vi "Plucker_Force_CoordTransform.vi"(9 "R_{1}_{2}":dbl[][](array[numeric]), 10 "d_{1}_{2} (mm)":dbl[](array[numeric]), 11 "F_{1}":dbl[](array[numeric])) -> (3 "F_{2}":dbl[](array[numeric]))   [LabVIEW 2019]
uses:
  <vilib>/imath/engines/lvmath2/RunTimeEngine/Managers/WorkSpace/UID Generator.vi
  <vilib>/imath/engines/lvmath2/RunTimeEngine/BuiltInFunctions/size/NIMS_[I32,I32]=size(GRow).vi
  <instcachedir>/0/NIMS_[I32,I32]=size(GRow)_CFE2C4BDC5BC45CD88F2F6A295A2273D.lvgen/NIMS_[I32,I32]=size(GRow)_CFE2C4BDC5BC45CD88F2F6A295A2273D_001.vi
  <vilib>/imath/engines/lvmath2/RunTimeEngine/RunTimeType/NIMS_RunTimeType_From StrictType (excl LVString).vi
  <instcachedir>/0/NIMS_RunTimeType_From StrictType (excl LVString)_D8AFBA86A94845AAA577C895450664BD.lvgen/NIMS_RunTimeType_From StrictType (excl LVString)_D8AFBA86A94845AAA577C895450664BD_000.vi
  <vilib>/imath/engines/lvmath2/RunTimeEngine/LocalVariableDefStatement/MC_LocalVariableDefStatement_Display.vi
  <vilib>/imath/engines/lvmath2/RunTimeEngine/IndexRead/NIMS V(S).vi
  <instcachedir>/0/NIMS V(S)_0488751826AF41519A22953C041130DC.lvgen/NIMS V(S)_0488751826AF41519A22953C041130DC_000.vi
  <vilib>/imath/engines/lvmath2/RunTimeEngine/ErrorHandling/NIMS_Create Error From Enums.vi
  <vilib>/imath/engines/lvmath2/RunTimeEngine/RowToken/NIMS_RowToken_M_M.vi
  <instcachedir>/0/NIMS_RowToken_M_M_21FE36D058524603B8B587AC30FD72C2.lvgen/NIMS_RowToken_M_M_21FE36D058524603B8B587AC30FD72C2_004.vi
  <vilib>/imath/engines/lvmath2/RunTimeEngine/ArithmeticOperatorToken/NIMS_ArithmeticOperator_multmx.vi
  <instcachedir>/0/NIMS_ArithmeticOperator_multmx_77F1D2D6F4D94BA7A97C4E7185C02392.lvgen/NIMS_ArithmeticOperator_multmx_77F1D2D6F4D94BA7A97C4E7185C02392_004.vi
  <vilib>/imath/engines/lvmath2/RunTimeEngine/MatrixToken/NIMS_MatrixToken_M_M.vi
  <instcachedir>/0/NIMS_MatrixToken_M_M_5CE23C568F32465C96BE328F7823DCA0.lvgen/NIMS_MatrixToken_M_M_5CE23C568F32465C96BE328F7823DCA0_004.vi
  <vilib>/imath/engines/lvmath2/RunTimeEngine/BuiltInFunctions/inv/NIMS_inv(GM).vi
  <instcachedir>/0/NIMS_inv(GM)_A6DF8FE880224208AACFE4CF9F659502.lvgen/NIMS_inv(GM)_A6DF8FE880224208AACFE4CF9F659502_000.vi
  <vilib>/imath/engines/lvmath2/RunTimeEngine/ErrorHandling/NIMS_Error From Error Code.vi
  <vilib>/imathl/engines/lvmath/Functions/Error Handling/Create Error.vi
  <vilib>/imath/engines/lvmath2/RunTimeEngine/Managers/SymbolTable/Clear UID.vi
  <vilib>/imath/engines/lvmath2/RunTimeEngine/NodeEndStatement/NIMS_NodeEndStatement_Output.vi
  <instcachedir>/0/NIMS_NodeEndStatement_Output_53EC0D466D134D7ABD903AC30B43404B.lvgen/NIMS_NodeEndStatement_Output_53EC0D466D134D7ABD903AC30B43404B_002.vi
  <vilib>/imath/engines/lvmath2/RunTimeEngine/ErrorHandling/NIMS_Finalize Error.vi
  <vilib>/imath/engines/lvmath2/RunTimeEngine/Managers/SymbolTable/NIMS_WorkSpace.lvlib
panel:
  out "X":dbl[][](array[numeric])
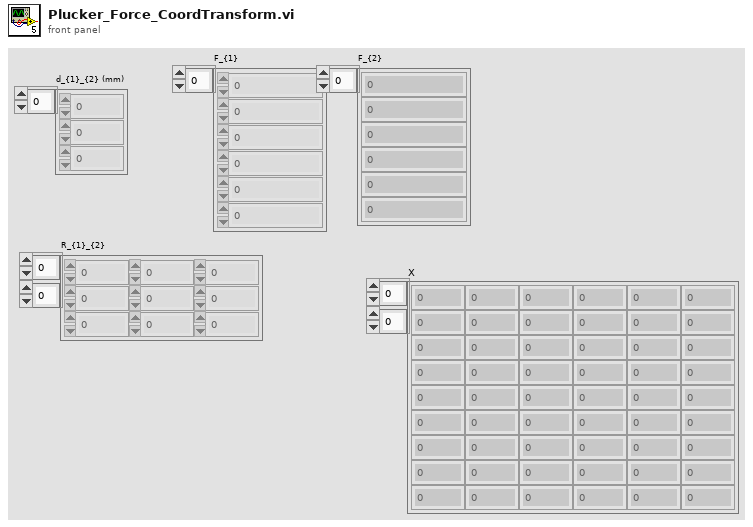
[diagram p1: front panel]
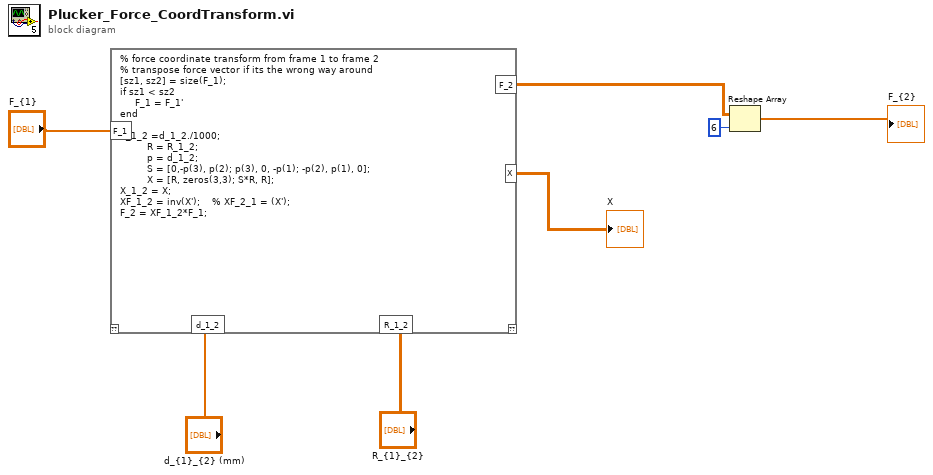
[diagram p0: block diagram]
diagram:
  n1 = mathscript code="% force coordinate transform from frame 1 to frame 2 \n% transpose force vector if its the wrong way around\n[sz1, sz2] = size(F_1);\nif sz1 < sz2\n     F_1 = F_1'\nend\n\nd_1_2 =d_1_2./1000;\n         R = R_1_2;\n         p = d_1_2;\n         S = [0,-p(3), p(2); p(3), 0, -p(1); -p(2), p(1), 0];\n         X = [R, zeros(3,3); S*R, R]; \nX_1_2 = X;\nXF_1_2 = inv(X');    % XF_2_1 = (X');\nF_2 = XF_1_2*F_1;"("F_1"="F_{1}", "d_1_2"="d_{1}_{2} (mm)", "R_1_2"="R_{1}_{2}") -> ("F_2"=w4:dbl[][], "X"=→"X":dbl[][])  [unwired: 1 in, 1 out]
  n2 = Reshape Array(w4, 6 ("dimension size")) -> (→"F_{2}":dbl[])
